vi "Trial Based Experiment Runner.vi"(11 "Experiment":refnum<class "TrialBasedExperiment.lvclass">) -> ()   [LabVIEW 2010, in "Core SubVIs.lvlib"]
doc: "Use this template to measure or generate signals using the DAQ Assistant Express VI and NI-DAQmx. Double click the DAQ Assistant Express VI to launch a configuration wizard which steps you through configuring a measurement or generation.\n\nNote: You must have an NI-DAQmx compatible device installed to use this Express VI. Refer to the DAQ Quick Start Guide for NI-DAQ 7.0 for a list of compatible devices."
uses:
  Core SubVIs/Core SubVIs.lvlib
  Trial Based Experiment.lvsc/Inputs.ctl
  TrialBasedExperimentObject/TrialBasedExperiment.lvclass
  Trial Based Experiment.lvsc/Outputs.ctl
  Trial Based Experiment.lvsc/StatechartState.ctl
  Trial Based Experiment.lvsc/State.ctl
  Core SubVIs/Controls/TYPE - Analog Data Queue Method.ctl
  Core SubVIs/Controls/TYPE - Timer Control.ctl
  Trial Based Experiment.lvsc/Trigger.ctl
  <vilib>/Statechart/Nodes/EventFiring/NI_SC_EventFiringNode.xnode
  Trial Based Experiment.lvsc
  <vilib>/Statechart/Infrastructure/RTStatechart/RunTime SCN.xnode
  <vilib>/Statechart/Common/IntGuid.ctl
  <vilib>/Statechart/Common/DbgID.ctl
  Trial Based Experiment.lvsc/CompanionDiagram.vi/142/SC Main.vi
  HDF5/HDF5.lvlib
  Program Files/National Instruments/LabVIEW 2010/resource/objmgr/daqmx.rc
  <vilib>/Statechart/Common/NI_SC_LVSCCommonFiles.lvlib
panel:
  out "Timeout":dbl
  out "Active States":T1
  in  "Subject":string(combo)="Ben"
  out "Recording Path":path
  out "Missed Updates":dbl
  out "Fixated":bool
  in  "Optical Track Var":refnum<k21>="\\\\localhost\\SharedVariable\\EyeTrace"
  in  "Optical Tracker":bool
  out "State machine":i32
  out "Events":i32
  out "Data processing":i32
  in  "Squirt Time(ms)":u32=50
  out "Hammer clock":bool=TRUE
  in  "Pause":bool
  out "Terminated?":bool
  in  "Bad Stop!":bool
  in  "Stop":bool=TRUE
  in  "Juice":bool
  out "Outputs":T3
  out "State machine inputs":T4={"Timing"={"Intertrial time"=2000.0, "Acquire fixation time"=1234.0, "Hold fixation time"=2000.0, "Delay period time"=2000.0, "Response time"=2000.0, "Reward"=100.0, "Punish time"=1500.0}, "Stop"=FALSE, "Control states"={"Fixated"=FALSE, "Centered"=FALSE}, "Pause"=FALSE, "Hammer running"=TRUE, "Experiment"=refnum}
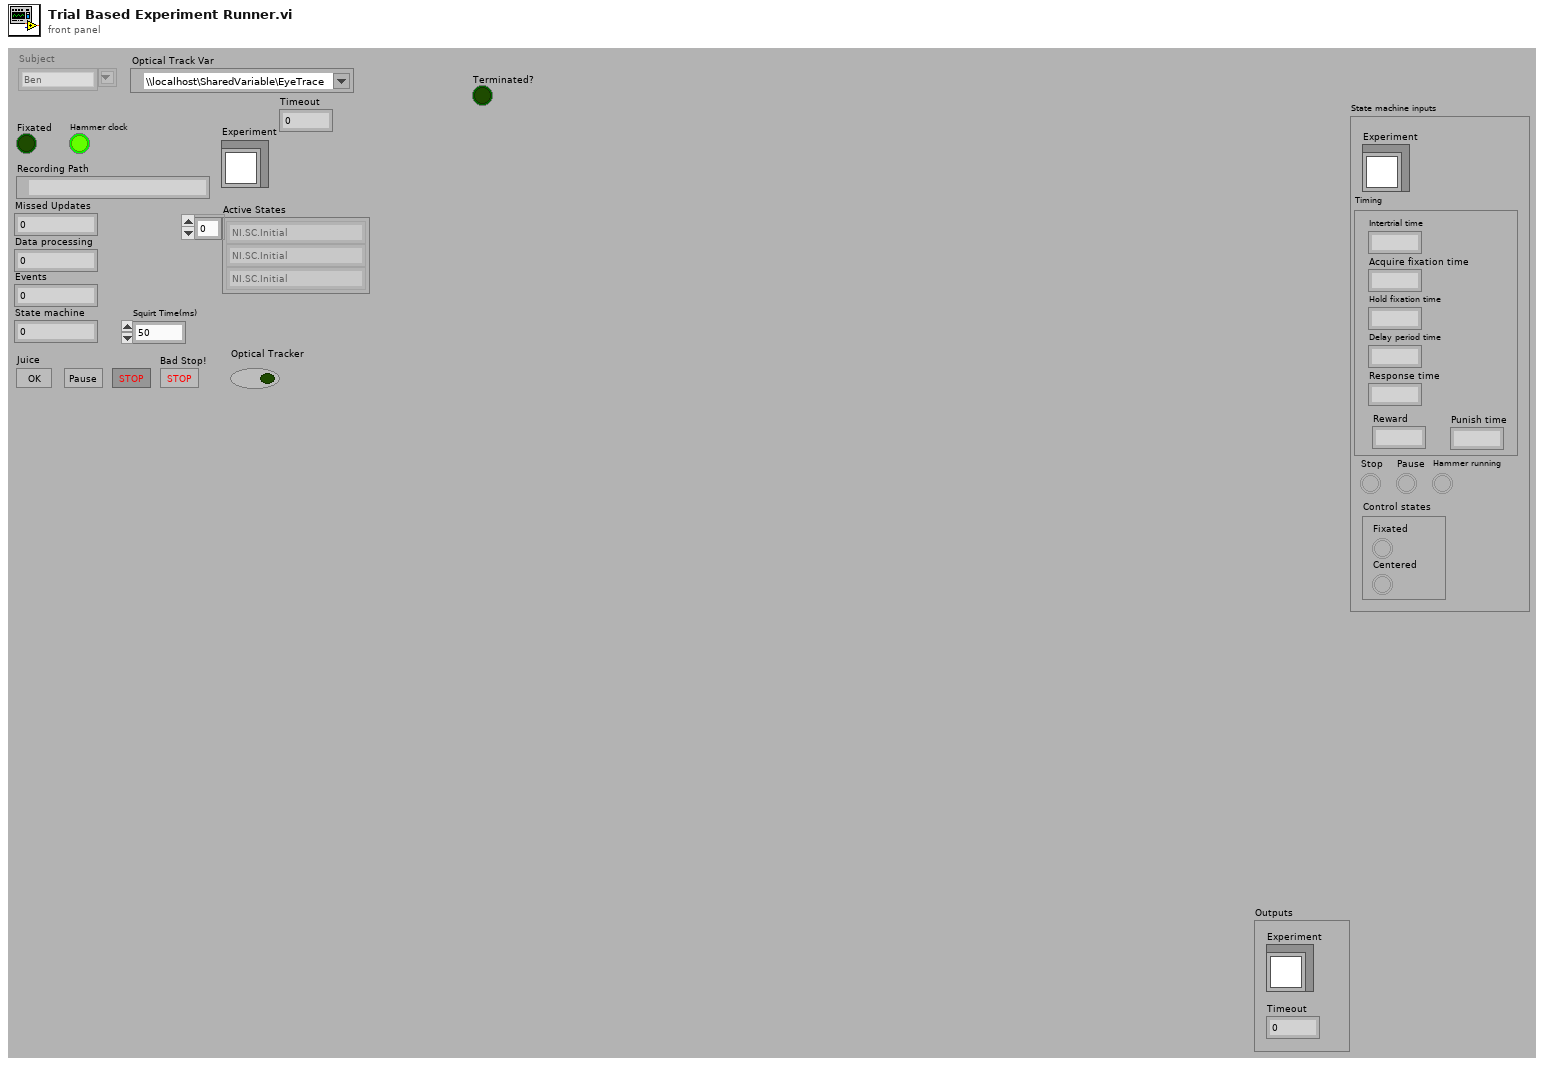
[diagram p1: front panel]
types:
  T1 = typedef "Trial Based Experiment.lvsc/StatechartState.ctl" = T2[]
  T2 = typedef "Trial Based Experiment.lvsc/State.ctl" = enum16{"NI.SC.Initial", "NI.SC.History", "NI.SC.ShallowHistory", "NI.SC.Terminal", "Running", "Cleanup", "Running\\Region\\Pause", "Running\\Region\\Response Period", "Running\\Region\\Delay Period", "Running\\Region\\Hold Fixation", "Running\\Region\\Acquire Fixation", "Running\\Region\\Abort Trial", "Running\\Region\\End Trial", "Running\\Region\\Intertrial", "Running\\Region\\Start Trial"}
  T3 = typedef "Trial Based Experiment.lvsc/Outputs.ctl" = cluster{"Experiment":refnum<class "TrialBasedExperiment.lvclass">, "Timeout":dbl}
  T4 = typedef "Trial Based Experiment.lvsc/Inputs.ctl" = cluster{"Timing":cluster{"Intertrial time":dbl, "Acquire fixation time":dbl, "Hold fixation time":dbl, "Delay period time":dbl, "Response time":dbl, "Reward":dbl, "Punish time":dbl}, "Stop":bool, "Control states":cluster{"Fixated":bool, "Centered":bool}, "Pause":bool, "Hammer running":bool, "Experiment":refnum<class "TrialBasedExperiment.lvclass">}
  T5 = typedef "Core SubVIs.lvlib/TYPE - Analog Data Queue Method.ctl" = enum16{"Set Data Queue", "Preview Element", "Remove Element", "Get Data Queue", "Flush Data Queue"}
  T6 = cluster{"sample rate":dbl, "actual sample rate":dbl, "frame size":dbl}
  T7 = cluster{"raw data cache size":u32, "raw data cache elements":i32, "meta data cache elements":i32, "w0":dbl}
  T8 = enum16{"Read", "Write", "ReadWrite", "BufferedRead", "BufferedReadWrite"}
  T9 = cluster{"file ID":i32, "dataset_id":i32, "offset":dbl, "timestamp_id":i32, "timestamp_offset":dbl}
  T10 = typedef "Core SubVIs.lvlib/TYPE - Named Data Structures.ctl" = cluster{"Loop Name (DAQ Loop)":string, "queue out":refnum<queue>, "FileSettings":cluster{"file ID":i32, "dataset_id":i32, "offset":dbl, "timestamp_id":i32, "timestamp_offset":dbl}}
  T11 = typedef "Core SubVIs.lvlib/TYPE - Timer Control.ctl" = enum16{"Reset Timer", "Read Timer"}
  T12 = typedef "Trial Based Experiment.lvsc/Trigger.ctl" = enum16{"NULL", "Fixated", "Broke Fixation", "Stop", "Correct Response", "Incorrect Response", "Timeout"}
  T13 = typedef "Core SubVIs.lvlib/TYPE - Analog Data.ctl" = waveform(dbl)[]
  T14 = typedef "NI_SC_LVSCCommonFiles.lvlib/IntGuid.ctl" = cluster{"Data1":u32, "Data2":u16, "Data3":u16, "Data4":u8, "Data5":u8, "Data6":u8, "Data11":u8, "Data9":u8, "Data10":u8, "Data8":u8, "Data7":u8}
  T15 = typedef "NI_SC_LVSCCommonFiles.lvlib/DbgID.ctl" = cluster{"VIRef":u32, "IntGUID":T14}
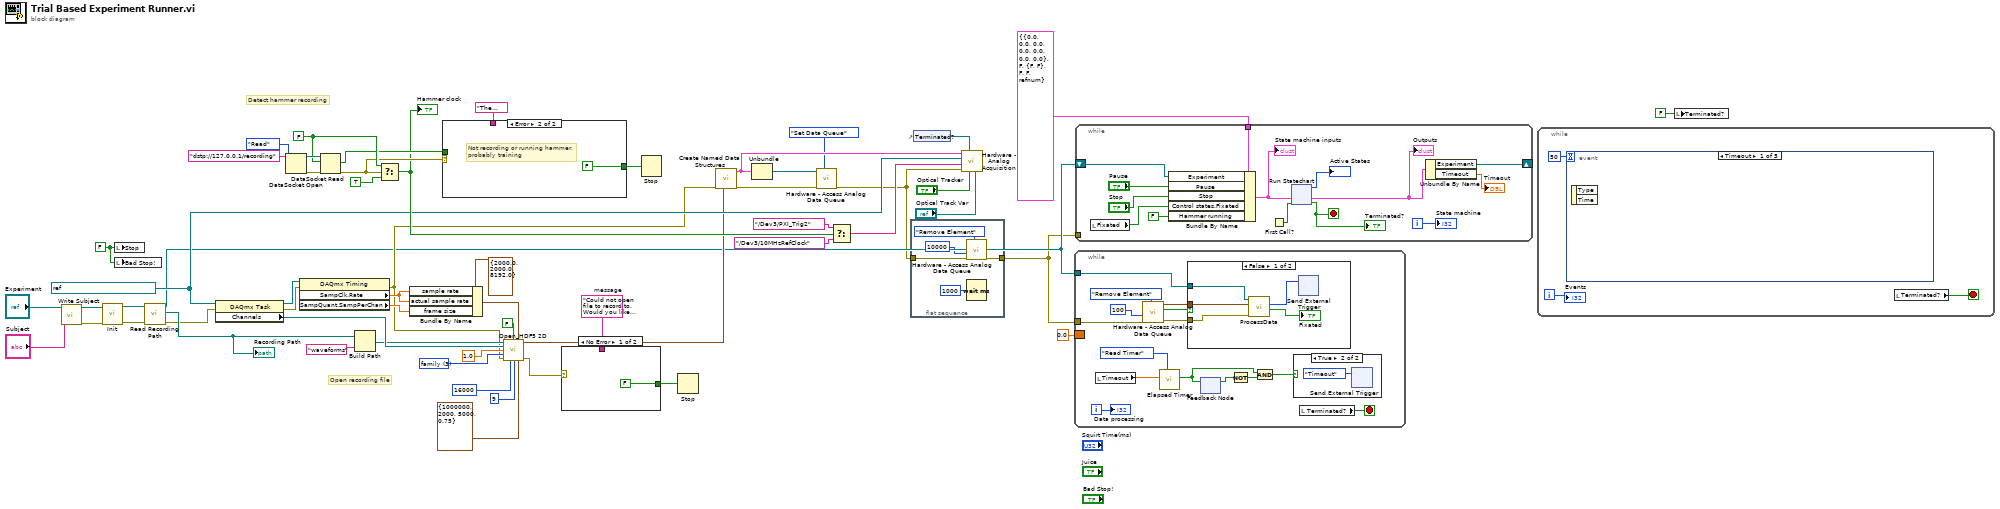
[diagram p0: block diagram]
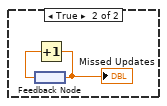
[diagram p3: hidden frame]
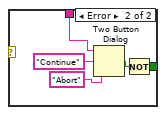
[diagram p4: hidden frame]
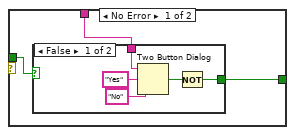
[diagram p5: hidden frame]
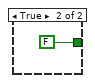
[diagram p6: hidden frame]
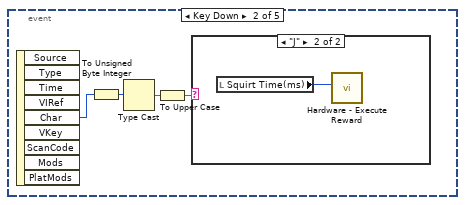
[diagram p7: hidden frame]
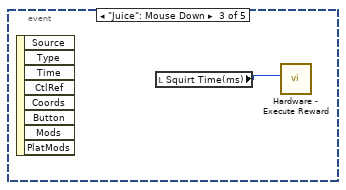
[diagram p9: hidden frame]
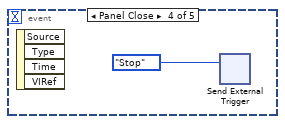
[diagram p10: hidden frame]
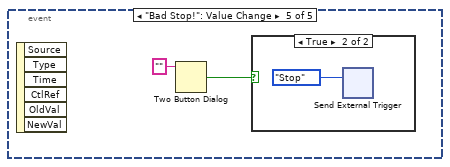
[diagram p11: hidden frame]
diagram:
  w18 = FALSE ("stop")
  w22 = "Could not open file to record to.  Would you like to continue?"  # message
  w32 = u16 3 items=["sec2", "stdio", "split", "family"] ("driver")
  w49 = FALSE
  w37 = refnum<k21> "State System Analog Input" ("task/channels in")
  # "Detect hammer recording"
  # "Open recording file"
  n1 = call-dynamic "Write Subject.vi"("Subject"="Subject", "TrialBasedExperiment in"="Experiment") -> ("error out"=w2:errorcluster, "TrialBasedExperiment out"=w3:refnum<class "TrialBasedExperiment.lvclass">)  [unwired: 8 in]
  n2 = call-dynamic "Init.vi"("error in (no error)"=w2, "TrialBasedExperiment in"=w3) -> ("error out"=w15:errorcluster, "TrialBasedExperiment out"=w13:refnum<class "TrialBasedExperiment.lvclass">)  [unwired: 8 in]
  n3 = local write "Stop"(w18) -> ()
  n4 = local write "Bad Stop!"(w18) -> ()
  n5 = call-dynamic "Read Recording Path.vi"("error in (no error)"=w15, "TrialBasedExperiment in"=w13) -> ("error out"=w10:errorcluster, "Recording Path"=w36:path, "TrialBasedExperiment out"=w7:refnum<class "TrialBasedExperiment.lvclass">)  [unwired: 7 in]
  "Recording Path" <- w36
  n6 = property class="DAQmx Task"(reference=w37, error in=w10) -> (reference out=w11:refnum<k21>, error out=w12:errorcluster, "Channels"=w24:refnum<k21>[])
  n7 = DataSocket Open(10:T8."Read" ("mode"), 11:"dstp://127.0.0.1/recording" ("URL")) -> (0:w52:errorcluster, 3:w51:refnum<k13>)  [unwired: 1 in, 1 out]
  n8 = property class="DAQmx Timing"(reference=w11, error in=w12) -> (error out=w9:errorcluster, "SampClk.Rate"=w27:dbl, "SampQuant.SampPerChan"=w25:dbl)  [unwired: 1 out]
  n9 = DataSocket Read(8:w52, 10:w49, 11:w51) -> (0:w45:errorcluster, 2:w48:bool)  [unwired: 7 out]
  n10 = Build Path(base path=w36, name or relative path="waveforms") -> (appended path=w20:path)
  n11 = Select(t=w49, s=w45, f=TRUE) -> (s? t:f=w40:bool)
  "Hammer clock" <- w40
  n12 = Bundle By Name(cluster=T6 {"sample rate"=2000.0, "actual sample rate"=2000.0, "frame size"=8192.0} ("sampling info"), "sample rate"=w27, "actual sample rate"=w27, "frame size"=w25) -> (w26:T6)
  n13 = case shown="Error" w45 {
    tunnel: w48 -> [w60 _]
    tunnel: "The hammer recording socket appears to exist, but is false.  This means you have hammer running but are not recording any data.  Do you want to continue?" ("message") -> [w59 _]
    tunnel: [w58 FALSE ("T button?")] -> w46
    frame No Error {
      n14 = case shown="False" w60 {
        tunnel: w59 -> [w65 _]
        tunnel: [w61 FALSE ("T button?")] -> w58
        frame False {
          n15 = Two Button Dialog(message=w65, 1:"No" ("F button name (\"Cancel\")"), 2:"Yes" ("T button name (\"OK\")")) -> (T button?=w62:bool)
          n16 = Not(x=w62) -> (.not. x?=w61:bool)
        }
        frame True {
        }
      }
    }
    frame Error {
      # "Not recording or running hammer,\nprobably training"
    }
  }
  n17 = call "Open_HDF5 2D.vi"("filename"=w20, "Compress"=FALSE ("compress?"), "sampling info"=w26, "channel names"=w24, "gain"=1.0, "driver"=w32, "error in"=w9, "chunk length"=u32 16000 ("chunk length rows"), "level"=9, "cache specs"=T7 {"raw data cache size"=1000000, "raw data cache elements"=2000, "meta data cache elements"=5000, "w0"=0.75}) -> ("output cluster"=w14:T9, "error out"=w23:errorcluster)  [unwired: 1 in, 3 out]
  n18 = case shown="No Error" w23 {
    tunnel: w22 -> [_ w73]
    tunnel: [FALSE w69] -> w21
    frame No Error {
    }
    frame Error {
      n19 = Two Button Dialog(message=w73, 1:"Abort" ("F button name (\"Cancel\")"), 2:"Continue" ("T button name (\"OK\")")) -> (T button?=w70:bool)
      n20 = Not(x=w70) -> (.not. x?=w69:bool)
    }
  }
  n21 = Stop(stop? (T)=w46) -> ()
  n22 = Stop(stop? (T)=w21) -> ()
  n23 = call "Create Named Data Structures.vi"("FileSettings"=w14, "error in (no error)"=w9) -> ("error out"=w17:errorcluster, "Named Data Structures"=w57:T10)  [unwired: 3 in, 5 out]
  n24 = Unbundle(w57) -> ("queue out"=w16:refnum<queue>)  [unwired: 2 out]
  n25 = call "Hardware - Access Analog Data Queue.vi"("Method"=TYPE_-_Analog_Data_Queue_Method."Set Data Queue", "error in (no error)"=w17, "Analog Data Queue"=w16) -> ("error out"=w6:errorcluster)  [unwired: 1 in, 7 out]
  n26 = Select(t=tag "/Dev3/PXI_Trig2" ("Clock Base"), s=w40, f=tag "/Dev3/10MHzRefClock" ("Clock Base")) -> (s? t:f=w55:tag)
  n27 = flat-sequence {
    tunnel: w6 -> [w76]
    tunnel: [w75] -> w5
    frame #0 {
      n28 = call "Hardware - Access Analog Data Queue.vi"("Method"=TYPE_-_Analog_Data_Queue_Method."Remove Element", "error in (no error)"=w76, "timeout in ms (-1)"=10000) -> ("error out"=w75:errorcluster)  [unwired: 1 in, 7 out]
      n29 = Wait (ms)(milliseconds to wait=u32 1000) -> ()  [unwired: 1 out]
    }
  }
  n30 = control-ref of="Terminated?"() -> (w42:refnum<vi>)
  n31 = call "Hardware - Analog Acquisition.vi"("Shared Variable Control"="Optical Track Var", "Optical Tracker"="Optical Tracker", "Terminated?"=w42, "error in"=w6, "SampClk.Timebase.Src"=w55, "task/channels in"=w37, "Named Data Structures"=w57) -> ()  [unwired: 5 out]
  n32 = while {
    tunnel: w5 -> [w91]
    tunnel: w7 -> [w89]
    border: 0.0 -> [_]
    i -> [w87]
    stop <- w90 stop-if-true
    n33 = local read "Timeout"() -> (w83:dbl)
    n34 = call "Hardware - Access Analog Data Queue.vi"("Method"=TYPE_-_Analog_Data_Queue_Method."Remove Element", "error in (no error)"=w91, "timeout in ms (-1)"=100) -> ("error out"=w85:errorcluster, "timed out?"=w86:bool, "Analog Data"=w88:T13)  [unwired: 1 in, 5 out]
    n35 = call "Elapsed Timer.vi"("Timer Control"=TYPE_-_Timer_Control."Read Timer", "Timeout (ms)"=w83) -> ("Time Elapsed?"=w80:bool)  [unwired: 7 in, 2 out]
    n36 = case shown="False" w86 {
      tunnel: w89 -> [w115 _]
      tunnel: w88 -> [w114 _]
      tunnel: w85 -> [w111 _]
      frame False {
        n37 = call-dynamic "ProcessData.vi"("error in (no error)"=w111, "Analog Data"=w114, "TrialBasedExperiment in"=w115) -> ("Fixated"=→"Fixated":bool, "Trigger"=w113:T12)  [unwired: 5 in, 2 out]
        n38 = xnode "Send External Trigger"("Trigger"=w113) -> ()  [unwired: 1 in, 2 out]
      }
      frame True {
        n39 = feedback #1() -> (w132:dbl)
        n40 = Increment(x=w132) -> (x+1=w133:dbl)
        "Missed Updates" <- w133
        n41 = feedback-in #1(w133) -> ()
      }
    }
    n42 = feedback-in #2(w80) -> ()
    n43 = feedback #2() -> (w82:bool)  [unwired: 1 in]
    n44 = Not(x=w82) -> (.not. x?=w81:bool)
    n45 = And(x=w80, y=w81) -> (x .and. y?=w79:bool)
    n46 = case shown="True" w79 {
      frame False {
      }
      frame True {
        n47 = xnode "Send External Trigger"("Trigger"=Trigger."Timeout") -> ()  [unwired: 1 in, 2 out]
      }
    }
    n48 = local read "Terminated?"() -> (w90:bool)
    "Data processing" <- w87
  }
  n49 = while {
    tunnel: w5 -> [_]
    tunnel: T4 {"Timing"={"Intertrial time"=0.0, "Acquire fixation time"=0.0, "Hold fixation time"=0.0, "Delay period time"=0.0, "Response time"=0.0, "Reward"=0.0, "Punish time"=0.0}, "Stop"=FALSE, "Control states"={"Fixated"=FALSE, "Centered"=FALSE}, "Pause"=FALSE, "Hammer running"=FALSE, "Experiment"=refnum} ("Inputs") -> [w139]
    shift-right: [w137] -> _
    shift-left: w7 -> [w136]
    i -> [w145]
    stop <- w142 stop-if-true
    n50 = local read "Fixated"() -> (w143:bool)
    n51 = Bundle By Name(cluster=w139, "Experiment"=w136, "Pause"="Pause", "Stop"="Stop", "Control states.Fixated"=w143, "Hammer running"=FALSE) -> (w141:T4)
    "State machine inputs" <- w141
    n52 = First Call?() -> (First Call?: T/F=w144:bool)
    n53 = xnode "Run Statechart"("Init?"=w144, "Inputs"=w141) -> ("Terminated?"=w142:bool, "Outputs"=w138:T3, "Active States"=→"Active States":T1)
    "Outputs" <- w138
    "Terminated?" <- w142
    n54 = Unbundle By Name(w138) -> ("Experiment"=w137:refnum<class "TrialBasedExperiment.lvclass">, "Timeout"=→"Timeout":dbl)
    "State machine" <- w145
  }
  n55 = while {
    i -> [w239]
    stop <- w240 stop-if-true
    n56 = event shown="[0] Timeout" {
      selector: _ -> [_ _ _ _ _]
      dyn-events: _ -> [_ _ _ _ _]
      timeout: 50 -> [_ _ _ _ _]
      event Timeout {
        n57 = event-data() -> ()  [unwired: 3 out]
      }
      event Key Down {
        n58 = event-data() -> ("Char"=w245:i16)  [unwired: 9 out]
        n59 = To Unsigned Byte Integer(number=w245) -> (unsigned 8bit integer=w244:u8)
        n60 = Type Cast(x=w244) -> (*(type *) &x=w243:string)  [unwired: 1 out]
        n61 = To Upper Case(1:w243) -> (0:w242:string)
        n62 = case shown="\"J\"" w242 {
          frame "0", Default {
          }
          frame "J" {
            n63 = local read "Squirt Time(ms)"() -> (w246:u32)
            n64 = call "Hardware - Execute Reward.vi"("Reward Time (200 ms)"=w246) -> ()  [unwired: 1 in, 10 out]
          }
        }
      }
      event "Juice": Mouse Down {
        n65 = event-data() -> ()  [unwired: 9 out]
        n66 = local read "Squirt Time(ms)"() -> (w247:u32)
        n67 = call "Hardware - Execute Reward.vi"("Reward Time (200 ms)"=w247) -> ()  [unwired: 1 in, 10 out]
      }
      event Panel Close {
        n68 = event-data() -> ()  [unwired: 5 out]
        n69 = xnode "Send External Trigger"("Trigger"=Trigger."Stop") -> ()  [unwired: 1 in, 2 out]
      }
      event "Bad Stop!": Value Change {
        n70 = event-data() -> ()  [unwired: 7 out]
        n71 = Two Button Dialog(message="") -> (T button?=w265:bool)  [unwired: 2 out]
        n72 = case shown="True" w265 {
          frame False {
          }
          frame True {
            n73 = xnode "Send External Trigger"("Trigger"=Trigger."Stop") -> ()  [unwired: 1 in, 2 out]
          }
        }
      }
    }
    n74 = local read "Terminated?"() -> (w240:bool)
    "Events" <- w239
  }
  n75 = local write "Terminated?"(FALSE ("Terminated?")) -> ()
